vi "WSVCAP SHL FPGA LL Procedure I2C - Receive Byte.vi"(0 "Procedure Step":T1, 1 "Wait Ticks Remaining":u32, 5 "I2C Wait Ticks":u32, 7 "Read Bits Remaining":u8, 9 "Read Bytes Remaining":u8, 11 "error in (no error)":errorcluster, 13 "Socket Mask":u64 format="%012x") -> (3 "Wait Ticks Remaining Out":u32, 4 "Procedure Step Out":T1, 6 "Finished":bool, 8 "Read Bits Remaining Out":u8, 10 "Read Bytes Remaining Out":u8, 15 "error out":errorcluster)   [LabVIEW 2012]
uses:
  Type Defs/WSVCAP SHL Procedure Step Enum.ctl
  Type Defs/WSVCAP SHL I2C Write Line Enum.ctl
  Type Defs/WSVCAP SHL FIFO Operation Enum.ctl
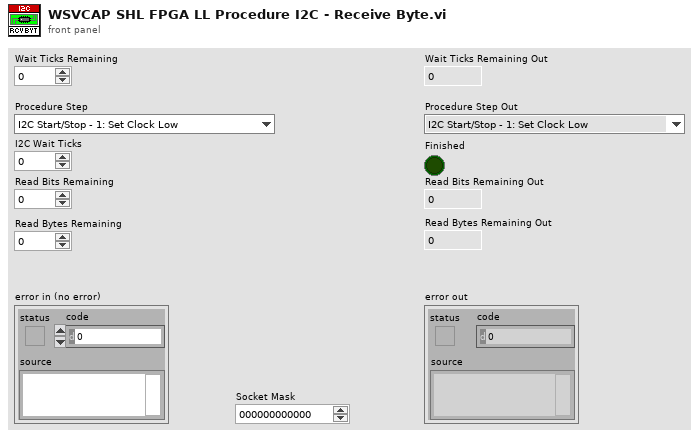
[diagram p1: front panel]
types:
  T1 = typedef "WSVCAP SHL Procedure Step Enum.ctl" = enum16{"I2C Start/Stop - 1: Set Clock Low", "I2C Start/Stop - 2: Wait", "I2C Start/Stop - 3: Set Data I", "I2C Start/Stop - 4: Wait", "I2C Start/Stop - 5: Set Clock High", "I2C Start/Stop - 6: Wait", "I2C Start/Stop - 7: Set Data II", "I2C Start/Stop - 8: Wait", "I2C Start/Stop - 9: Set Clock Low", "I2C Start/Stop - 10: Wait", "I2C Read ACK - 1: Set Clock High", "I2C Read ACK - 2: Wait", "I2C Read ACK - 3: Read ACK Bit", "I2C Read ACK - 4: Wait", "I2C Read ACK - 5: Set Clock Low", "I2C Read ACK - 6: Wait", "I2C Write ACK - 1: Write ACK Bit", "I2C Write ACK - 2: Wait", "I2C Write ACK - 3: Set Clock High", "I2C Write ACK - 4: Wait", "I2C Write ACK - 5: Set Clock Low", "I2C Write ACK - 6: Wait", "I2C Write ACK - 7: Set Data Low", "I2C Send Add - 1: Reset Bits Remaining", "I2C Send Add - 2: Set Data Bit", "I2C Send Add - 3: Wait", "I2C Send Add - 4: Set Clock High", "I2C Send Add - 5: Wait", "I2C Send Add - 6: Set Clock Low", "I2C Send Add - 7: Wait", "I2C Send Add - 8: Check Bits Remaining", "I2C Send Data - 1: Reset Bits Remaining", "I2C Send Data - 2: Load Write Bit from FIFO", "I2C Send Data - 3: Set Data Bit", "I2C Send Data - 4: Wait", "I2C Send Data - 5: Set Clock High", "I2C Send Data - 6: Wait", "I2C Send Data - 7: Set Clock Low", "I2C Send Data - 8: Wait", "I2C Send Data - 9: Check Bits Remaining", "I2C Receive Data - 1: Reset Bits Remaining", "I2C Receive Data - 2: Wait", "I2C Receive Data - 3: Set Clock High", "I2C Receive Data - 4: Wait", "I2C Receive Data - 5: Read Data Bit", "I2C Receive Data - 6: Wait", "I2C Receive Data - 7: Set Clock Low", "I2C Receive Data - 8: Wait", "I2C Receive Data - 9: Check Bits Remaining", "SPI Clear Lines - 1:Clear", "SPI Send/Receive - 1: Load SDA - Clock Low", "SPI Send/Receive - 2: Wait", "SPI Send/Receive - 3: Load DATO - Clock High", "SPI Send/Receive - 4: Wait", "SPI Wait CMD Delay - 1:Wait", "RFFE Send SSC - 1:Set Low", "RFFE Send SSC - 2:Wait", "RFFE Send SSC - 3:Set SDA High", "RFFE Send SSC - 4:Wait", "RFFE Send SSC - 5:Set SDA Low", "RFFE Send SSC - 6:Wait", "RFFE Send Data - 1:Set SCL High", "RFFE Send Data - 2:Wait", "RFFE Send Data - 3:Set SCL Low", "RFFE Send Data - 4:Wait", "RFFE Send Data - 5:Set SCL High (P)", "RFFE Send Data - 6:Wait", "RFFE Send Data - 7:Set SCL Low (P)", "RFFE Send Data - 8:Wait", "RFFE Send Data - 9:Set SCL High (BP)", "RFFE Send Data - 10:Wait", "RFFE Send Data - 11:Set SCL Low (BP)", "RFFE Send Data - 12:Wait", "RFFE Receive Data - 1:Set SCL High", "RFFE Receive Data - 2:Wait", "RFFE Receive Data - 3:Set SCL Low", "RFFE Receive Data - 4:Wait", "RFFE Receive Data - 5:Set SCL High (BP)", "RFFE Receive Data - 6:Wait", "RFFE Receive Data - 7:Set SCL Low (BP)", "RFFE Receive Data - 8:Wait", "RFFE Wait CMD Delay - 1:Wait", "RFFE Clear Lines - 1:Clear"}
  T2 = typedef "WSVCAP SHL I2C Write Line Enum.ctl" = enum16{"I2C SCL", "I2C SDA"}
  T3 = typedef "WSVCAP SHL FIFO Operation Enum.ctl" = enum16{"Create FIFO/Memory", "Get Write FIFO Status", "Get Read FIFO Status", "Put Element in Write", "Put Element in Read", "Get Element from Write", "Get Element from Read"}
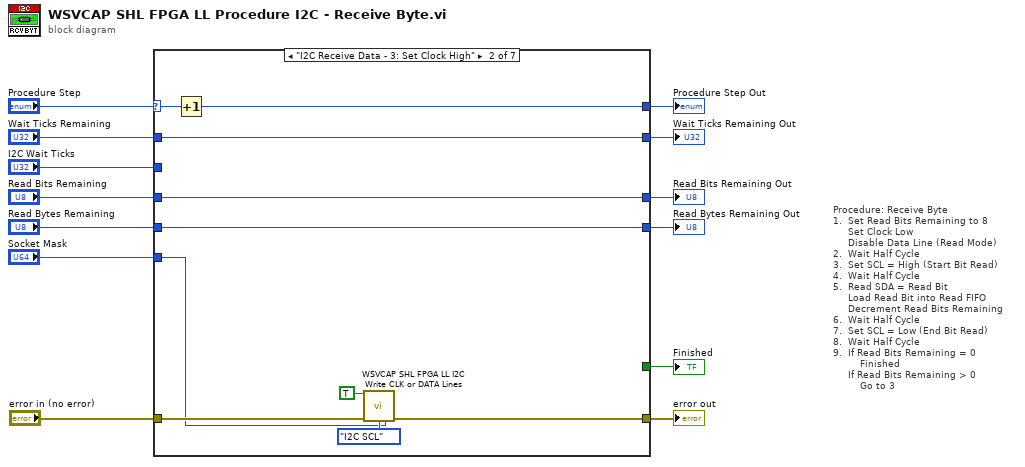
[diagram p0: block diagram]
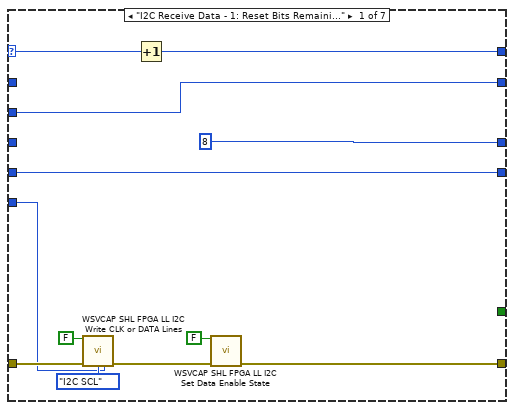
[diagram p2: hidden frame]
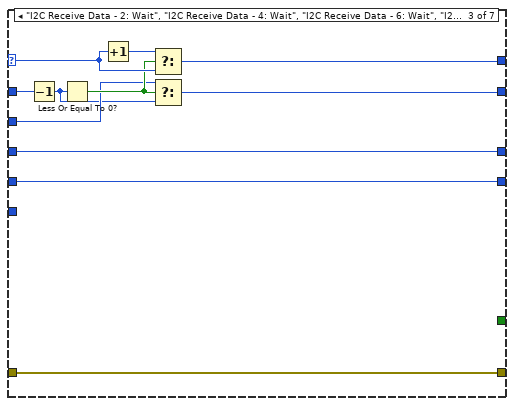
[diagram p3: hidden frame]
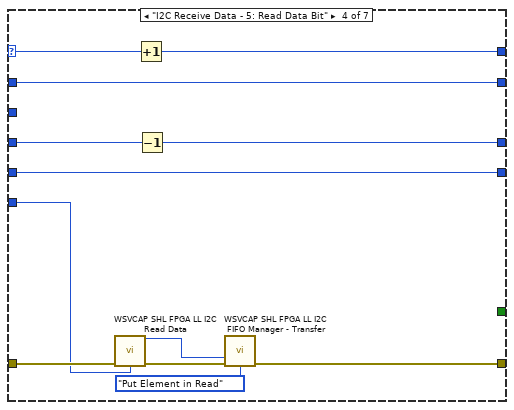
[diagram p4: hidden frame]
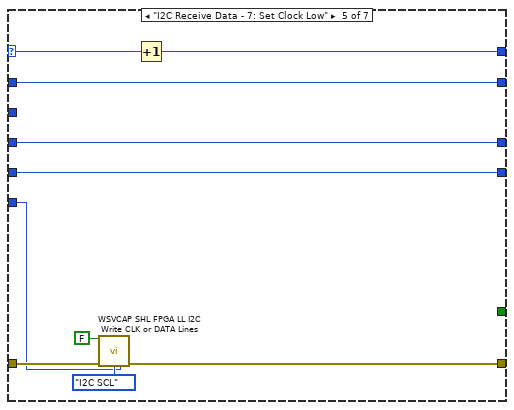
[diagram p5: hidden frame]
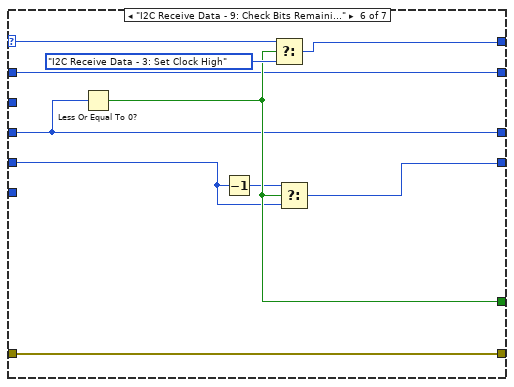
[diagram p6: hidden frame]
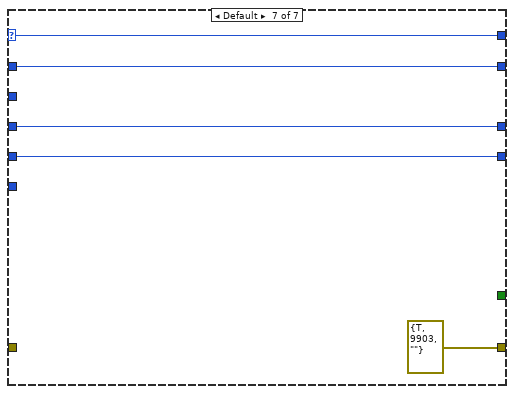
[diagram p7: hidden frame]
diagram:
  # "Procedure: Receive Byte\n1.  Set Read Bits Remaining to 8 \n     Set Clock Low\n     Disable Data Line (Read Mode)\n2.  Wait Half Cycle\n3.  Set SCL = High (Start Bit Read)\n4.  Wait Half Cycle\n5.  Read SDA = Read Bit\n     Load Read Bit into Read FIFO\n     Decrement Read Bits Remaining\n6.  Wait Half Cycle\n7.  Set SCL = Low (End Bit Read)\n8.  Wait Half Cycle\n9.  If Read Bits Remaining = 0\n         Finished\n     If Read Bits Remaining > 0\n         Go to 3"
  n1 = case shown="\"I2C Receive Data - 3: Set Clock High\"" "Procedure Step" {
    selector: "Procedure Step" -> [w22 w32 w45 w57 w64 w73 w82]
    tunnel: [w20 w33 w43 w55 w66 w78 errorcluster {"status"=TRUE, "code"=9903, "source"=""} ("error IO")] -> w12
    tunnel: "error in (no error)" -> [w24 w34 w43 w58 w67 w78 _]
    tunnel: "Wait Ticks Remaining" -> [_ w28 w46 w48 w61 w70 w81]
    tunnel: "I2C Wait Ticks" -> [w15 _ w41 _ _ _ _]
    tunnel: "Read Bits Remaining" -> [_ w27 w37 w52 w60 w69 w80]
    tunnel: [_ _ _ _ _ w76 _] -> w11
    tunnel: "Socket Mask" -> [w18 w30 _ w51 w63 _ _]
    tunnel: "Read Bytes Remaining" -> [w14 w26 w36 w47 w59 w75 w79]
    tunnel: [w17 w29 w39 w50 w62 w72 w82] -> w10
    tunnel: [w14 w26 w36 w47 w59 w71 w79] -> w9
    tunnel: [w15 w28 w38 w48 w61 w70 w81] -> w2
    tunnel: [u8 8 ("Write Bits Remaining") w27 w37 w49 w60 w69 w80] -> w1
    frame "I2C Receive Data - 1: Reset Bits Remaining" {
      n2 = call "WSVCAP SHL FPGA LL I2C Write CLK or DATA Lines.vi"("Bit In"=FALSE, "error in (no error)"=w24, "Line"=WSVCAP_SHL_I2C_Write_Line_Enum."I2C SCL", "Socket Mask"=w18) -> ("error out"=w21:errorcluster)  [unwired: 11 in]
      n3 = Increment(x=w22) -> (x+1=w17:T1)
      n4 = call "WSVCAP SHL FPGA LL I2C Set Data Enable State.vi"("State"=FALSE, "error in (no error)"=w21) -> ("error out"=w20:errorcluster)  [unwired: 13 in]
    }
    frame "I2C Receive Data - 3: Set Clock High" {
      n5 = Increment(x=w32) -> (x+1=w29:T1)
      n6 = call "WSVCAP SHL FPGA LL I2C Write CLK or DATA Lines.vi"("Bit In"=TRUE, "error in (no error)"=w34, "Line"=WSVCAP_SHL_I2C_Write_Line_Enum."I2C SCL", "Socket Mask"=w30) -> ("error out"=w33:errorcluster)  [unwired: 11 in]
    }
    frame "I2C Receive Data - 2: Wait", "I2C Receive Data - 4: Wait", "I2C Receive Data - 6: Wait", "I2C Receive Data - 8: Wait" {
      n7 = Decrement(x=w46) -> (x-1=w40:u32)
      n8 = Less Or Equal To 0?(x=w40) -> (x <= 0?=w42:bool)
      n9 = Increment(x=w45) -> (x+1=w44:T1)
      n10 = Select(t=w44, s=w42, f=w45) -> (s? t:f=w39:T1)
      n11 = Select(t=w41, s=w42, f=w40) -> (s? t:f=w38:u32)
    }
    frame "I2C Receive Data - 5: Read Data Bit" {
      n12 = call "WSVCAP SHL FPGA LL I2C Read Data.vi"("error in (no error)"=w58, "Socket Mask"=w51) -> ("Long Word Out (1-Bit for Each Channel)"=w53:u64, "error out"=w56:errorcluster)  [unwired: 12 in]
      n13 = Increment(x=w57) -> (x+1=w50:T1)
      n14 = Decrement(x=w52) -> (x-1=w49:u8)
      n15 = call "WSVCAP SHL FPGA LL I2C FIFO Manager - Transfer.vi"("Long Word In"=w53, "error in (no error)"=w56, "Operation"=WSVCAP_SHL_FIFO_Operation_Enum."Put Element in Read") -> ("error out"=w55:errorcluster)  [unwired: 10 in, 2 out]
    }
    frame "I2C Receive Data - 7: Set Clock Low" {
      n16 = call "WSVCAP SHL FPGA LL I2C Write CLK or DATA Lines.vi"("Bit In"=FALSE, "error in (no error)"=w67, "Line"=WSVCAP_SHL_I2C_Write_Line_Enum."I2C SCL", "Socket Mask"=w63) -> ("error out"=w66:errorcluster)  [unwired: 11 in]
      n17 = Increment(x=w64) -> (x+1=w62:T1)
    }
    frame "I2C Receive Data - 9: Check Bits Remaining" {
      n18 = Less Or Equal To 0?(x=w69) -> (x <= 0?=w76:bool)
      n19 = Decrement(x=w75) -> (x-1=w74:u8)
      n20 = Select(t=w73, s=w76, f=WSVCAP_SHL_Procedure_Step_Enum."I2C Receive Data - 3: Set Clock High" ("Procedure Step")) -> (s? t:f=w72:T1)
      n21 = Select(t=w74, s=w76, f=w75) -> (s? t:f=w71:u8)
    }
    frame Default {
    }
  }
  "error out" <- w12
  "Finished" <- w11
  "Procedure Step Out" <- w10
  "Read Bytes Remaining Out" <- w9
  "Wait Ticks Remaining Out" <- w2
  "Read Bits Remaining Out" <- w1
